vi "Timing-Get Reference Timestamp.vi"() -> (8 "double precision float":dbl format="%#_15g")   [LabVIEW 2020]
uses:
  <vilib>/Utility/miscctls.llb/LVDateTimeRec.ctl
panel:
  out "time stamp":timestamp
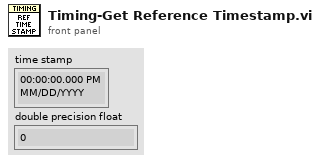
[diagram p1: front panel]
types:
  T1 = typedef "LVDateTimeRec.ctl" = cluster{"fractional second":dbl, "second":i32, "minute":i32, "hour":i32, "day of month":i32, "month":i32, "year":i32, "day of week":i32, "day of year":i32, "DST":i32}
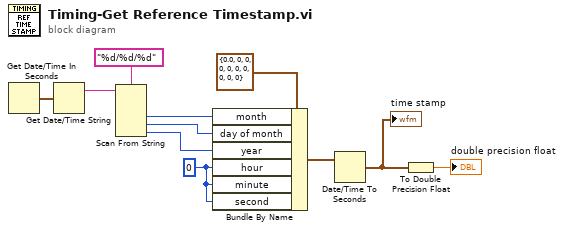
[diagram p0: block diagram]
diagram:
  w6 = 0 ("hour")
  n1 = Get Date/Time In Seconds() -> (seconds since 1Jan1904=w11:timestamp)
  n2 = Get Date/Time String(seconds (now)=w11) -> (date string=w9:string)  [unwired: 2 in, 1 out]
  n3 = Scan From String(format string="%d/%d/%d", input string=w9) -> (output 1=w5:i32, output 2=w4:i32, output 3=w3:i32)  [unwired: 5 in, 3 out]
  n4 = Bundle By Name(cluster=T1 {"fractional second"=0.0, "second"=0, "minute"=0, "hour"=0, "day of month"=0, "month"=0, "year"=0, "day of week"=0, "day of year"=0, "DST"=0} ("date time rec"), "month"=w5, "day of month"=w4, "year"=w3, "hour"=w6, "minute"=w6, "second"=w6) -> (w7:T1)
  n5 = Date/Time To Seconds(2:w7) -> (0:w2:timestamp)  [unwired: 1 in]
  "time stamp" <- w2
  n6 = To Double Precision Float(number=w2) -> (double precision float=→"double precision float":dbl)
